vi "UI.vi"(8 "error in (no error)":errorcluster, 11 "View in":refnum<class "View.lvclass">) -> (0 "error out":errorcluster, 3 "View out":refnum<class "View.lvclass">)   [LabVIEW 2020, in "Page1.lvlib" / "View.lvclass"]
uses:
  View.lvclass
  View.lvclass/View.ctl
  Controller/Controller.lvclass
panel:
  in  "Setting":u32
  out "Time (s)":u32
  in  "Main Test Folder":path
  # "Page1 UI"
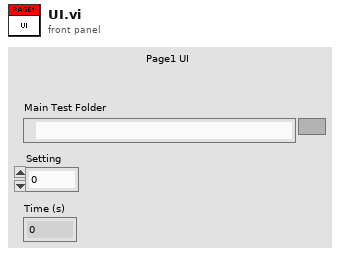
[diagram p1: front panel]
types:
  T1 = cluster{"Main Test Folder":refnum<vi>, "Time (s)":refnum<vi>, "Setting":refnum<vi>}
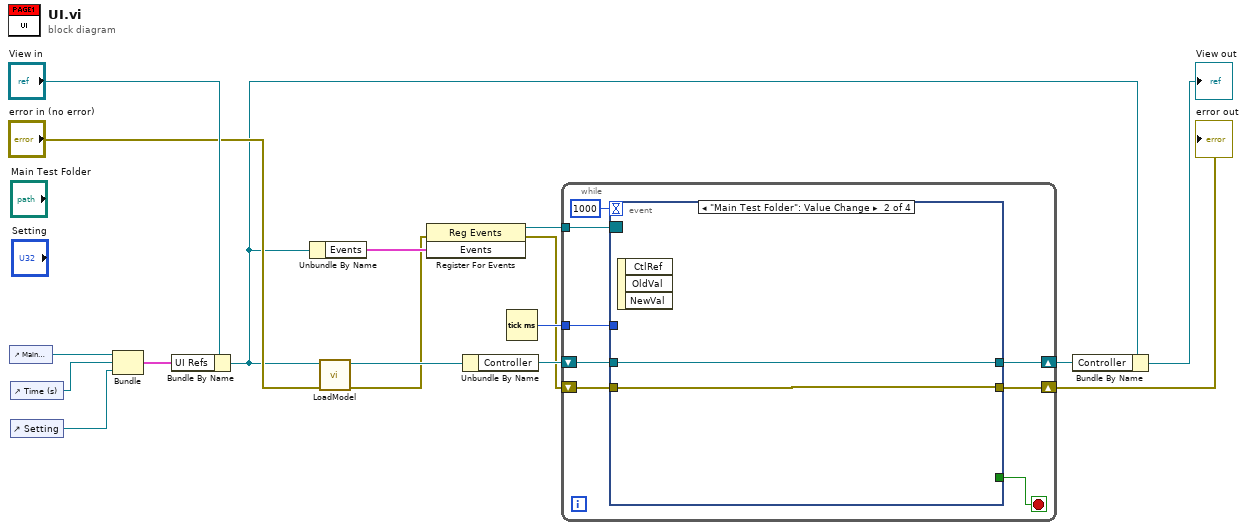
[diagram p0: block diagram]
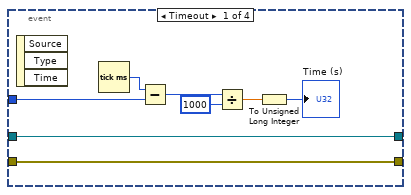
[diagram p2: hidden frame]
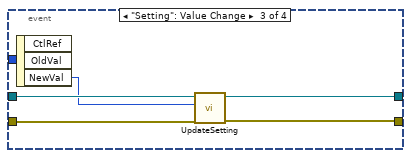
[diagram p3: hidden frame]
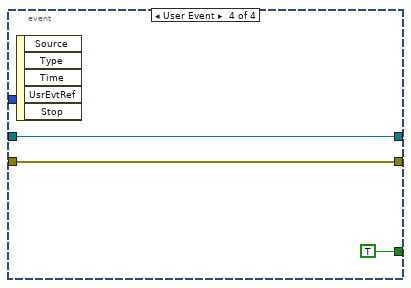
[diagram p4: hidden frame]
diagram:
  n1 = control-ref of="Main Test Folder"() -> (w14:refnum<vi>)
  n2 = control-ref of="Time (s)"() -> (w13:refnum<vi>)
  n3 = control-ref of="Setting"() -> (w6:refnum<vi>)
  n4 = Bundle("Main Test Folder"=w14, "Time (s)"=w13, "Setting"=w6) -> (w11:T1)  [unwired: 1 in]
  n5 = Bundle By Name(cluster="View in", "UI Refs"=w11) -> (w4:refnum<class "View.lvclass">)
  n6 = Unbundle By Name(w4) -> ("Events"=w17:cluster{"Stop":refnum<user-event>})
  n7 = call "LoadModel.vi"("error in (no error)"="error in (no error)", "View in"=w4) -> ("error out"=w7:errorcluster, "View out"=w9:refnum<class "View.lvclass">)  [unwired: 8 in]
  n8 = register-events(error in=w7, w17) -> (reference out=w16:refnum<event-registration>, error out=w1:errorcluster)  [unwired: 1 in]
  n9 = Unbundle By Name(w9) -> ("Controller"=w8:refnum<class "Controller.lvclass">)
  n10 = Tick Count (ms)() -> (millisecond timer value=w15:u32)
  n11 = while {
    tunnel: w16 -> [w25]
    tunnel: w15 -> [w22]
    shift-right: [w19] -> w5
    shift-left: w8 -> [w21]
    shift-right: [w18] -> w2
    shift-left: w1 -> [w20]
    stop <- w24 stop-if-true
    n12 = event shown="[1] \"Main Test Folder\": Value Change" {
      selector: w25 -> [_ _ _ _]
      dyn-events: _ -> [_ _ _ _]
      timeout: 1000 -> [_ _ _ _]
      tunnel: [_ _ _ TRUE] -> w24
      tunnel: w22 -> [w32 _ _ _]
      tunnel: w21 -> [w27 w35 w40 w42]
      tunnel: w20 -> [w26 w34 w38 w41]
      tunnel: [w27 w35 w39 w42] -> w19
      tunnel: [w26 w34 w37 w41] -> w18
      event Timeout {
        n13 = event-data() -> ()  [unwired: 1 in, 3 out]
        n14 = Tick Count (ms)() -> (millisecond timer value=w33:u32)
        n15 = Subtract(x=w33, y=w32) -> (x-y=w31:u32)
        n16 = Divide(x=w31, y=u32 1000) -> (x/y=w30:dbl)
        n17 = To Unsigned Long Integer(number=w30) -> (unsigned 32bit integer=→"Time (s)":u32)
      }
      event "Main Test Folder": Value Change {
        n18 = event-data() -> ()  [unwired: 1 in, 3 out]
      }
      event "Setting": Value Change {
        n19 = event-data() -> ("NewVal"=w36:u32)  [unwired: 1 in, 2 out]
        n20 = call "UpdateSetting.vi"("error in (no error)"=w38, "Setting"=w36, "Controller in"=w40) -> ("error out"=w37:errorcluster, "Controller out"=w39:refnum<class "Controller.lvclass">)  [unwired: 7 in]
      }
      event User Event {
        n21 = event-data() -> ()  [unwired: 1 in, 5 out]
      }
    }
  }
  "error out" <- w2
  n22 = Bundle By Name(cluster=w4, "Controller"=w5) -> (→"View out":refnum<class "View.lvclass">)
